vi "Automatic Dummy Epoxy Placement.vi"() -> ()   [LabVIEW 2021]
uses:
  Classes/Assembly/Assembly Run.lvclass
  Classes/Assembly/Database Entry/Database Entry.lvclass
  <vilib>/Utility/file.llb/Read Delimited Spreadsheet (string).vi
  SubVIs/PUT_region.vi
  SubVIs/component_tray_region.vi
  SubVIs/assembly_tray_region.vi
  Classes/Controller/I-O/I-O.lvclass
  Classes/Controller/Controller.lvclass
panel:
  in  "Abort assembly":bool
  in  "Do old-style single-module data-entry?":bool
  out "Status":string
  out "Stack names":T1
  out "Feet check":bool
  out "Assembly Type":string
  out "Assembly tray region":dbl
  out "Component tray region":dbl
  out "PUT Region":dbl
  # "Click the Run arrow to start.\nFill out pop-up prompts.\nSee Status for more info.\nAnswer ALL prompts until program stops running!"
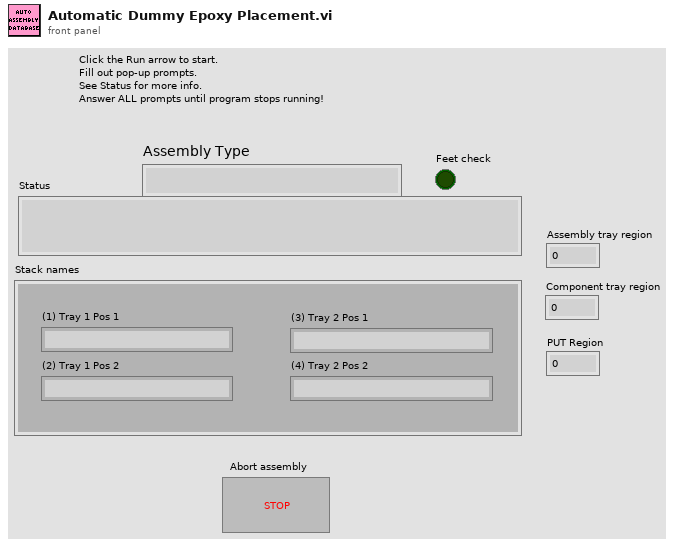
[diagram p1: front panel]
types:
  T1 = cluster{"(1) Tray 1 Pos 1":string, "(2) Tray 1 Pos 2":string, "(3) Tray 2 Pos 1":string, "(4) Tray 2 Pos 2":string}
  T2 = typedef "Controller.lvclass/Controllers.ctl" = cluster{"I-O.lvclass":refnum<class "I-O.lvclass">, "Gantry":refnum<k24>, "Dispenser":refnum<visa-resource-name>}
  T3 = typedef "File Paths.ctl" = cluster{"Glue Pattern Folder":path, "Carrier Tray Folder":path, "Pick Up Tool Fixture Folder":path, "Components Folder":path, "Bellows Tool Offset.txt":path, "Pick Up Tool Offset.txt":path, "Dispense Tip Offset.txt":path, "Log Files":path, "Gantry Assembly Map.txt":path, "Syringe and offset map.txt":path, "Controllers Folder":path, "Local dbase config":path}
  T4 = cluster{"Fixture ID":dbl, "Position":dbl, "Thickness":dbl}[]
  T5 = cluster{"Fixture ID":dbl, "Position":dbl, "Thickness":dbl}[][]
  T6 = cluster{"Stack names[0]":string, "Stack names[1]":string, "Stack names[2]":string, "Stack names[3]":string}
  T7 = cluster{"Fixture ID":dbl, "Position":dbl, "Thickness":dbl}
  T8 = typedef "I-O.lvclass/Pin Map.ctl" = cluster{"Region Valves":i32[], "Extra Valves":dbl[][][], "Tool Primary Valve":i32, "Tool Secondary Valve":i32, "Region Sensors":i32[], "Extra Sensors":dbl[][][], "Tool Primary Sensor":dbl, "Tool Secondary Sensor":dbl, "Compression Sensor":dbl, "5V":i32, "Dispenser Sensor":dbl, "Light Curtain":i32}
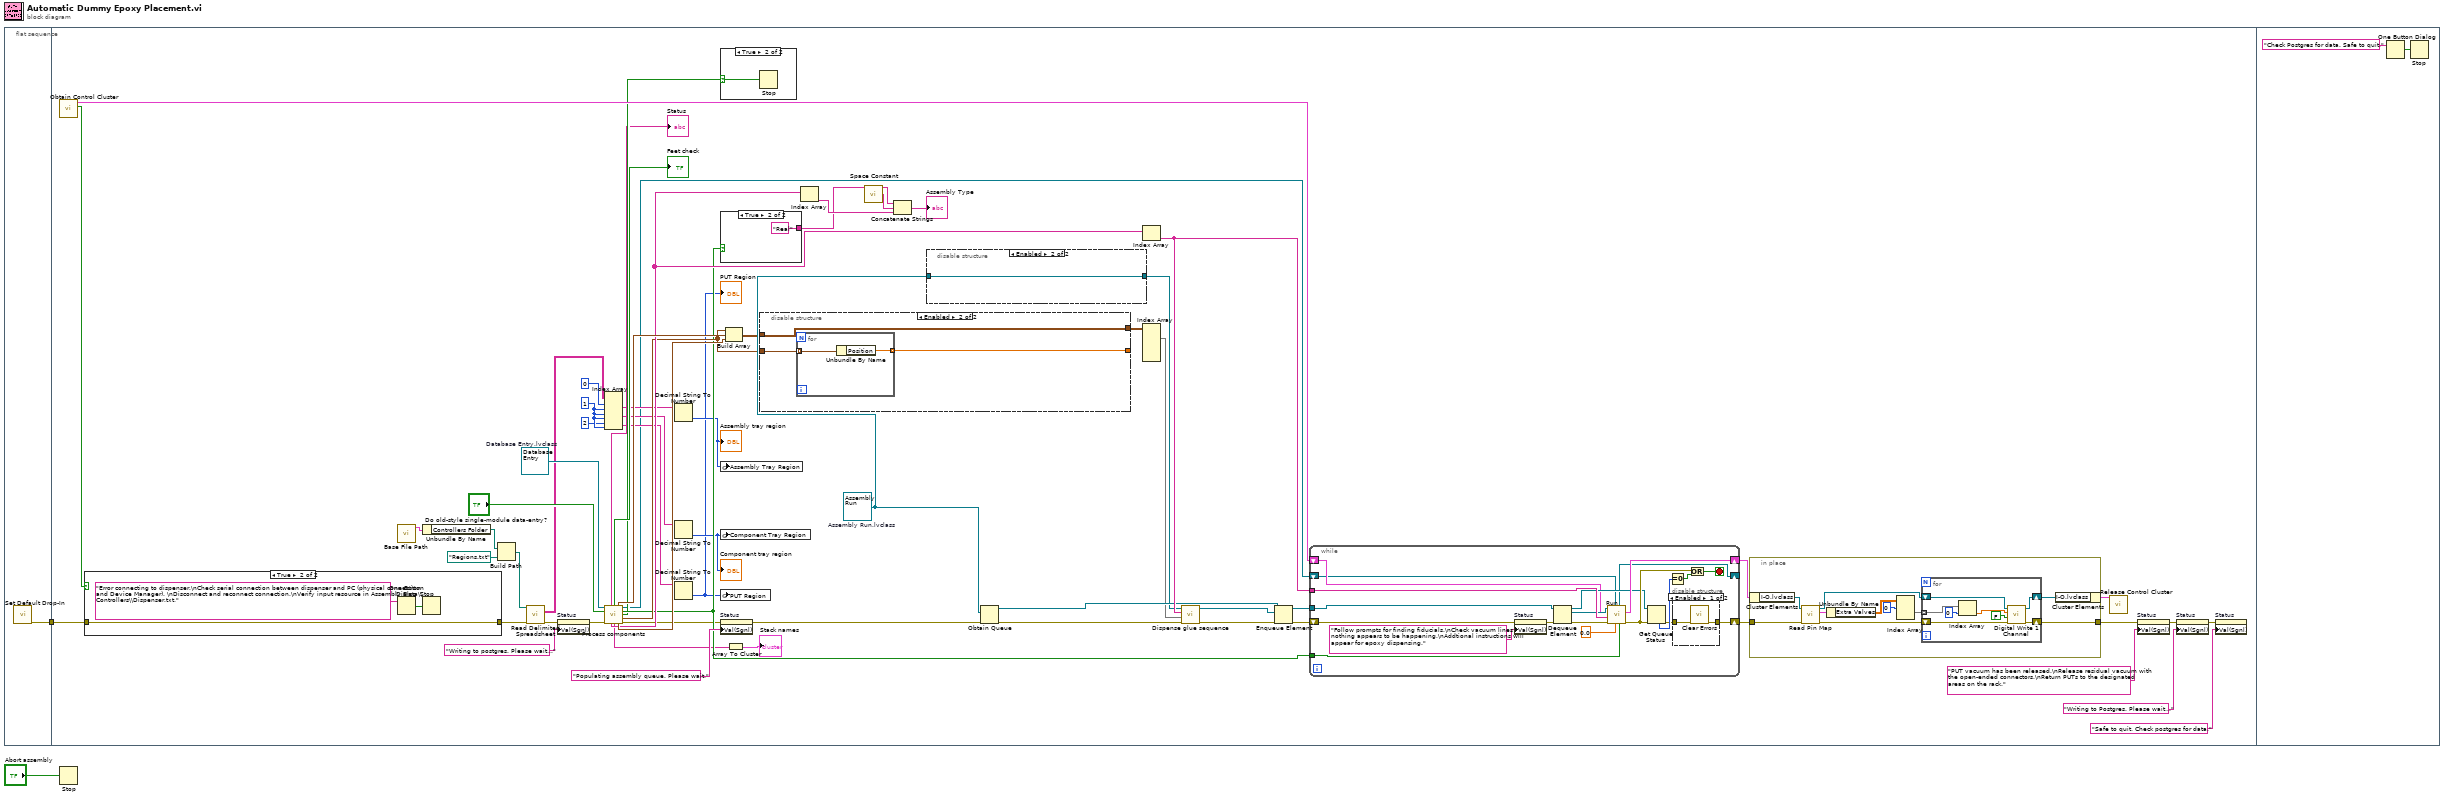
[diagram p0: block diagram]
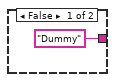
[diagram p3: hidden frame]
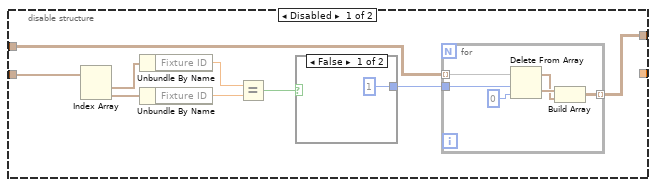
[diagram p5: hidden frame]
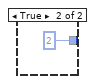
[diagram p6: hidden frame]
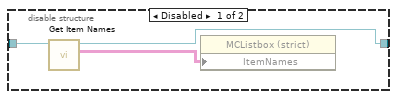
[diagram p7: hidden frame]
diagram:
  n1 = flat-sequence {
    tunnel: [w3] -> w2
    tunnel: w2 -> [w15]
    frame #0 {
      n2 = call "Set Default Drop-In.vi"() -> ("error out"=w3:errorcluster)  [unwired: 11 in]
    }
    frame #1 {
      w20 = 1 ("disabled index (col)")
      w43 = refnum<class "Database Entry.lvclass"> refnum  # Database Entry.lvclass
      w65 = refnum<class "Assembly Run.lvclass"> refnum  # Assembly Run.lvclass
      n3 = call "Obtain Control Cluster.vi"() -> ("Dispenser error?"=w32:bool, "Control Out"=w58:T2)  [unwired: 10 in]
      n4 = case shown="True" w32 {
        tunnel: w15 -> [w84 w85]
        tunnel: [w84 w85] -> w14
        frame False {
        }
        frame True {
          n5 = One Button Dialog(message="Error connecting to dispenser.\nCheck serial connection between dispenser and PC (physical connection and Device Manager). \nDisconnect and reconnect connection.\nVerify input resource in Assembly Data\\Controllers\\Dispenser.txt.") -> (true=w86:bool)  [unwired: 1 in]
          n6 = Stop(stop? (T)=w86) -> ()
        }
      }
      n7 = call "Base File Path.vi"() -> ("Paths Out"=w31:T3)  [unwired: 11 in]
      n8 = Unbundle By Name(w31) -> ("Controllers Folder"=w29:path)
      n9 = Build Path(base path=w29, name or relative path=path "Regions.txt") -> (appended path=w30:path)
      n10 = call-poly <vilib>:"Read Delimited Spreadsheet.vi"("file path (dialog if empty)"=w30, "error in (no error)"=w14) -> ("all rows"=w18:string[][], "error out"=w16:errorcluster)  [unwired: 8 in, 4 out]
      n11 = property on="Status" class="Str"(error in=w16, "Val(Sgnl)"="Writing to postgres. Please wait..." ("Value (Signaling)")) -> (error out=w33:errorcluster)  [unwired: 1 in, 1 out]
      n12 = Index Array(array=w18, index (row) #1=0 ("index (row)"), index (col) #1=w20, index (row) #2=w20, index (col) #2=w20, index (row) #3=2 ("disabled index (row)"), index (col) #3=w20) -> (element #1=w23:string, element #2=w22:string, element #3=w24:string)
      n13 = call "Process components.vi"("Database Entry in"=w43, "Do single-module data entry?"="Do old-style single-module data-entry?", "error in (no error)"=w33) -> ("Status"=→"Status":string, "Feet check"=→"Feet check":bool, "PUT Settings"=w63:T4, "Database Entry out"=w4:refnum<class "Database Entry.lvclass">, "Is real run?"=w49:bool, "Aborted"=w40:bool, "Assembly Settings"=w59:T4, "Assembly Type"=w62:string[], "Stack names"=w42:string[], "Component Settings"=w64:T4, "error out"=w45:errorcluster)  [unwired: 1 in, 1 out]
      n14 = Decimal String To Number(string=w23) -> (number=w26:i32)  [unwired: 2 in, 1 out]
      "Assembly tray region" <- w26
      n15 = Decimal String To Number(string=w22) -> (number=w27:i32)  [unwired: 2 in, 1 out]
      "Component tray region" <- w27
      n16 = Decimal String To Number(string=w24) -> (number=w25:i32)  [unwired: 2 in, 1 out]
      "PUT Region" <- w25
      n17 = case shown="True" w40 {
        selector: w40 -> [_ w90]
        frame False {
        }
        frame True {
          n18 = Stop(stop? (T)=w90) -> ()
        }
      }
      n19 = case shown="True" w49 {
        tunnel: ["Dummy" "Real"] -> w35
        frame False {
        }
        frame True {
        }
      }
      n20 = global write "assembly_tray_region.vi" "Assembly Tray Region"(w26) -> ()
      n21 = global write "component_tray_region.vi" "Component Tray Region"(w27) -> ()
      n22 = global write "PUT_region.vi" "PUT Region"(w25) -> ()
      n23 = property on="Status" class="Str"(error in=w45, "Val(Sgnl)"="Populating assembly queue. Please wait." ("Value (Signaling)")) -> (error out=w44:errorcluster)  [unwired: 1 in, 1 out]
      n24 = Build Array(w59, w63, w64) -> (w55:T5)
      n25 = Array To Cluster(array=w42) -> (cluster=→"Stack names":T6)
      n26 = disable-structure shown="Enabled" {
        disable-tunnel: w59 -> [w99 w109]
        disable-tunnel: [w98 w110] -> w56
        disable-tunnel: w55 -> [w97 w110]
        disable-tunnel: [_ w108] -> _
        frame Disabled {
          n27 = Index Array(array=w99) -> (element #1=w96:T7, element #2=w95:T7)  [unwired: 2 in]
          n28 = Unbundle By Name(w96) -> ("Fixture ID"=w94:dbl)
          n29 = Unbundle By Name(w95) -> ("Fixture ID"=w93:dbl)
          n30 = Equal?(x=w94, y=w93) -> (x = y?=w92:bool)
          n31 = case shown="False" w92 {
            tunnel: [1 2] -> w91
            frame False {
            }
            frame True {
            }
          }
          n32 = for {
            tunnel: w97 -> [w107] mode=indexing
            tunnel: [w106] -> w98 mode=indexing
            tunnel: w91 -> [w102]
            n33 = Delete From Array(array=w107, length=w102, index=0) -> (deleted portion=w104:T4, array with subset deleted=w103:T4)
            n34 = Build Array(w104, w103) -> (w106:T5)
          }
        }
        frame Enabled {
          n35 = for {
            tunnel: w109 -> [w112] mode=indexing
            tunnel: [w111] -> w108 mode=indexing
            n36 = Unbundle By Name(w112) -> ("Position"=w111:dbl)
          }
        }
      }
      n37 = Index Array(array=w62) -> (element=w37:string)  [unwired: 1 in]
      n38 = call <vilib>:"Space Constant.vi"() -> ("String"=w36:string)
      n39 = Concatenate Strings(w35, w36, w37) -> (→"Assembly Type":string)
      n40 = disable-structure shown="Enabled" {
        disable-tunnel: w65 -> [w115 w116]
        disable-tunnel: [w113 w116] -> w57
        frame Disabled {
          n41 = call "Get Item Names.vi"("Assembly Run in"=w115) -> ("Item names"=w114:string[][], "Assembly Run out"=w113:refnum<class "Assembly Run.lvclass">)  [unwired: 8 in, 1 out]
          n42 = property class="MCListbox (strict)"("ItemNames"=w114) -> ()  [unwired: 2 in, 2 out]
        }
        frame Enabled {
        }
      }
      n43 = Obtain Queue(element data type=w65, error in (no error)=w44) -> (queue out=w60:refnum<queue>, error out=w46:errorcluster)  [unwired: 3 in, 1 out]
      n44 = Index Array(array=w62) -> (element=w61:string)  [unwired: 1 in]
      n45 = Index Array(array=w56) -> (element #1=w51:T4)  [unwired: 6 in, 2 out]
      n46 = call "Dispense glue sequence.vi"("error in (no error)"=w46, "Assembly Tray Settings Array"=w51, "Assembly Type"=w61, "Assembly Run in"=w57) -> ("error out"=w47:errorcluster, "Assembly Run out"=w52:refnum<class "Assembly Run.lvclass">)  [unwired: 6 in]
      n47 = Enqueue Element(queue=w60, element=w52, error in (no error)=w47) -> (queue out=w54:refnum<queue>, error out=w48:errorcluster)  [unwired: 1 in, 1 out]
      n48 = while {
        shift-right: [w136] -> w53
        shift-left: w58 -> [w120]
        tunnel: w61 -> [w135]
        tunnel: w54 -> [w134]
        tunnel: w49 -> [w130]
        shift-right: [w119] -> w13
        shift-left: w48 -> [w129]
        shift-right: [w117] -> _
        shift-left: w4 -> [w118]
        stop <- w132 stop-if-true
        n49 = property on="Status" class="Str"(error in=w129, "Val(Sgnl)"="Follow prompts for finding fiducials.\nCheck vacuum lines if nothing appears to be happening.\nAddtional instructions will appear for epoxy dispensing." ("Value (Signaling)")) -> (error out=w121:errorcluster)  [unwired: 1 in, 1 out]
        n50 = Dequeue Element(queue=w134, error in (no error)=w121) -> (queue out=w128:refnum<queue>, element=w125:refnum<class "Assembly Run.lvclass">, error out=w124:errorcluster)  [unwired: 1 in, 1 out]
        n51 = call-dynamic "Run.vi"("Dispense?"=w130, "Pickup_Test_Number"=0.0, "Database Entry in"=w118, "error in (no error)"=w124, "Assembly Type"=w135, "Control In"=w120, "Assembly In"=w125) -> ("error out"=w133:errorcluster, "Control Out"=w136:T2, "Database Entry out"=w117:refnum<class "Database Entry.lvclass">)  [unwired: 1 in, 1 out]
        n52 = Get Queue Status(queue=w128, error in (no error)=w133) -> (error out=w126:errorcluster, # elements in queue=w127:i32)  [unwired: 1 in, 6 out]
        n53 = Equal To 0?(x=w127) -> (x = 0?=w131:bool)
        n54 = disable-structure shown="Enabled" {
          disable-tunnel: w126 -> [w138 w139]
          disable-tunnel: [w137 w139] -> w119
          frame Enabled {
            n55 = call <vilib>:"Clear Errors.vi"("error in (no error)"=w138) -> ("error out"=w137:errorcluster)  [unwired: 5 in, 1 out]
          }
          frame Disabled {
          }
        }
        n56 = Or(x=w133, y=w131) -> (x .or. y?=w132:bool)
      }
      n57 = in-place {
        in-place-border: w13 -> [w68]
        in-place-border: [w66] -> w11
        n58 = in-place-cluster #1(w53) -> ("I-O.lvclass"=w70:refnum<class "I-O.lvclass">)
        n59 = call-dynamic "Read Pin Map.vi"("error in (no error)"=w68, "I-O in"=w70) -> ("error out"=w67:errorcluster, "Pin Map 2"=w75:T8, "I-O out"=w72:refnum<class "I-O.lvclass">)  [unwired: 7 in]
        n60 = Unbundle By Name(w75) -> ("Extra Valves"=w74:dbl[][][])
        n61 = Index Array(array=w74, index (dim 0)=0 ("index (page)")) -> (element=w73:dbl[][])  [unwired: 2 in]
        n62 = for {
          tunnel: w73 -> [w83] mode=indexing
          shift-right: [w81] -> w69
          shift-left: w72 -> [w82]
          shift-right: [w76] -> w66
          shift-left: w67 -> [w77]
          n63 = Index Array(array=w83, index=0) -> (element=w80:dbl)
          n64 = call-dynamic "Digital Write 1 Channel.vi"("error constant"=w77, "Value"=FALSE, "Channel"=w80, "I-O.lvclass"=w82) -> ("error IO"=w76:errorcluster, "I-O.lvclass 2"=w81:refnum<class "I-O.lvclass">)  [unwired: 6 in]
        }
        n65 = in-place-cluster #1("I-O.lvclass"=w69) -> (w10:T2)
      }
      n66 = call "Release Control Cluster.vi"("output cluster"=w10) -> ()  [unwired: 11 in]
      n67 = property on="Status" class="Str"(error in=w11, "Val(Sgnl)"="PUT vacuum has been released.\nRelease residual vacuum with the open-ended connectors.\nReturn PUTs to the designated areas on the rack." ("Value (Signaling)")) -> (error out=w9:errorcluster)  [unwired: 1 in, 1 out]
      n68 = property on="Status" class="Str"(error in=w9, "Val(Sgnl)"="Writing to Postgres. Please wait...") -> (error out=w8:errorcluster)  [unwired: 1 in, 1 out]
      n69 = property on="Status" class="Str"(error in=w8, "Val(Sgnl)"="Safe to quit. Check postgres for data.") -> ()  [unwired: 1 in, 2 out]
    }
    frame #2 {
      n70 = One Button Dialog(message="Check Postgres for data. Safe to quit.") -> (true=w141:bool)  [unwired: 1 in]
      n71 = Stop(stop? (T)=w141) -> ()
    }
  }
  n72 = Stop(stop? (T)="Abort assembly") -> ()
